vi "Automonous no shift 1 container.vi"() -> ()   [LabVIEW 2014]
uses:
  Autonomous 1 Container with Self Correction.ctl
  2015 Master Code RECYCLE RUSH/2015 Master Code RECYCLE RUSH/Robot Global Data.vi
  Desired Arm Position.vi
  <vilib>/Rock Robotics/WPI/RobotDrive/WPI_RobotDriveGetSetRefNum.vi
panel:
  in  "Cluster":T1
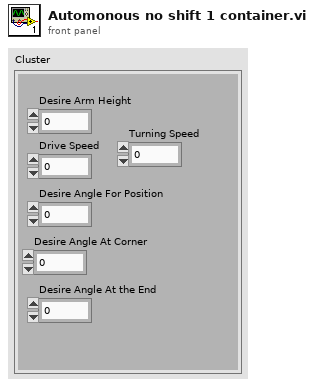
[diagram p1: front panel]
types:
  T1 = cluster{"Desire Arm Height":dbl, "Drive Speed":dbl, "Turning Speed":dbl, "Desire Angle At Corner ":dbl, "Desire Angle At the End":dbl, "Desire Angle For Position":dbl}
  T2 = typedef "Autonomous 1 Container with Self Correction.ctl" = enum16{"Start", "Pick Up Container", "Lift Container", "Drive To S.P", "Drive Straight", "Turn at Corner", "Move to Autozone", "Stop"}
  T3 = typedef "WPI_DigitalInputDevRef.ctl" = cluster{"DevStatus":errorcluster, "DIO Channel":T4, "Controller":T5}
  T4 = typedef "FPGA_DIOChannel.ctl" = enum8{"DIO 0", "DIO 1", "DIO 2", "DIO 3", "DIO 4", "DIO 5", "DIO 6", "DIO 7", "DIO 8", "DIO 9", "DIO MXP 0", "DIO MXP 1", "DIO MXP 2", "DIO MXP 3", "DIO MXP 4", "DIO MXP 5", "DIO MXP 6", "DIO MXP 7", "DIO MXP 8", "DIO MXP 9", "DIO MXP 10", "DIO MXP 11", "DIO MXP 12", "DIO MXP 13", "DIO MXP 14", "DIO MXP 15", "Invalid"}
  T5 = typedef "FPGA_TypedefDigitalModule.ctl" = enum16{"Controller 1"}
  T6 = typedef "WPI_RobotDriveDevRef.ctl" = cluster{"DevStatus":errorcluster, "Motors[]":T7[], "Square Inputs":bool, "Max Output":dbl}
  T7 = typedef "WPI_MotorControlDeviceRef.ctl" = cluster{"DeviceStatus":errorcluster, "Type":T8, "PWM":cluster{"Controller":T5, "PWM Channel":T9, "DeadBand":T10}, "CAN":cluster{"Device Number":u8, "Control Mode":T11, "Semaphore":T12, "Max Vout":dbl, "TalonSRX Control Mode":T13}, "Invert":bool, "TransformRef":T14, "InvTransformRef":T14}
  T8 = typedef "WPI_MotorControlType.ctl" = enum16{"PWM", "CAN", "CANTalonSRX"}
  T9 = typedef "FPGA_DIOPWMChannel.ctl" = enum8{"PWM 0", "PWM 1", "PWM 2", "PWM 3", "PWM 4", "PWM 5", "PWM 6", "PWM 7", "PWM 8", "PWM 9", "PWM MXP 0", "PWM MXP 1", "PWM MXP 2", "PWM MXP 3", "PWM MXP 4", "PWM MXP 5", "PWM MXP 6", "PWM MXP 7", "PWM MXP 8", "PWM MXP 9", "Invalid"}
  T10 = typedef "WPI_PWMDeadband.ctl" = cluster{"Name":string, "maxPositivePwm":i32, "minPositivePwm":i32, "centerPwm":i32, "maxNegativePwm":i32, "minNegativePwm":i32, "angularRange":u16}
  T11 = typedef "WPI_CANJaguar_ControlMode.ctl" = enum8{"Percent VBus", "Current", "Speed", "Position", "Voltage"}
  T12 = typedef "Semaphore RefNum" = refnum<k1>
  T13 = typedef "WPI_CANTalonSRX_APIControlMode.ctl" = enum8{"Percent VBus", "Speed", "Position", "Slave", "Unchanged / Invalid"}
  T14 = typedef "WPI_PWMTransform_ConPane.ctl" = refnum<vi>
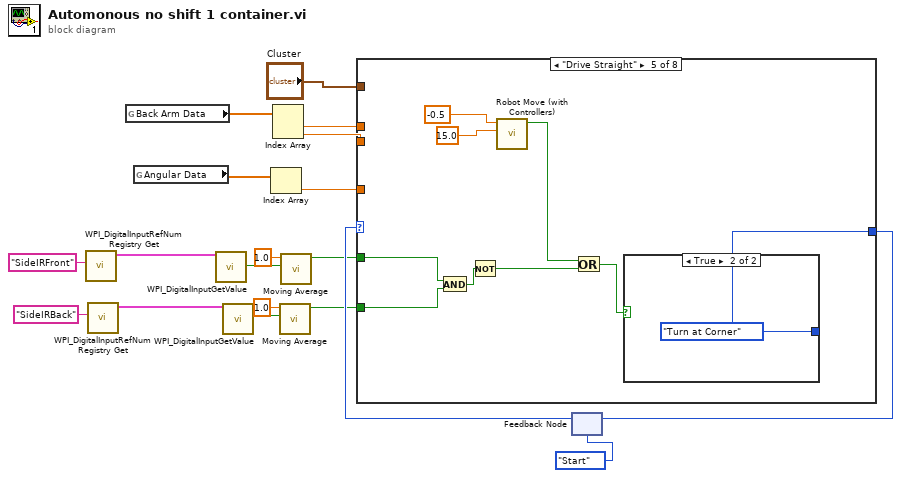
[diagram p0: block diagram]
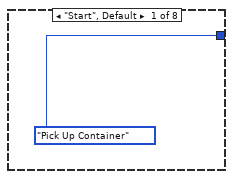
[diagram p2: hidden frame]
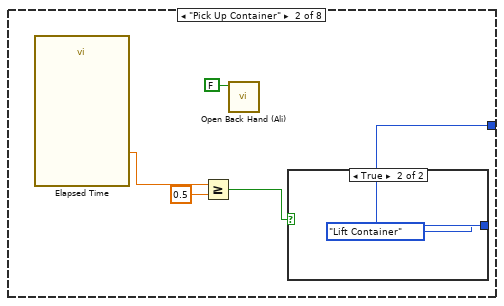
[diagram p3: hidden frame]
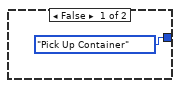
[diagram p4: hidden frame]
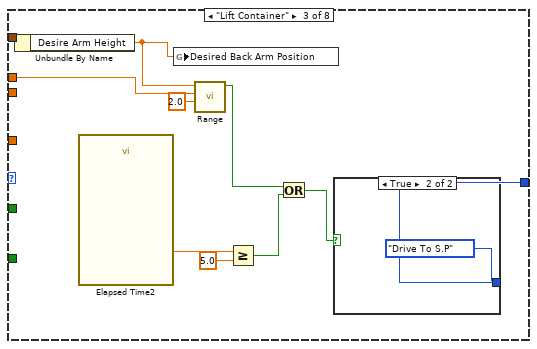
[diagram p5: hidden frame]
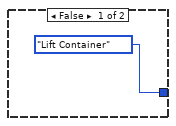
[diagram p6: hidden frame]
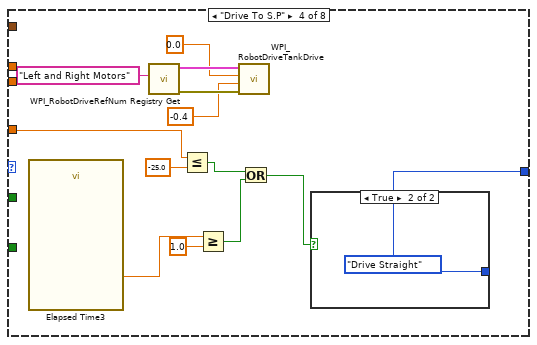
[diagram p7: hidden frame]
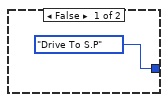
[diagram p8: hidden frame]
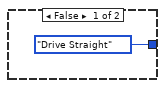
[diagram p9: hidden frame]
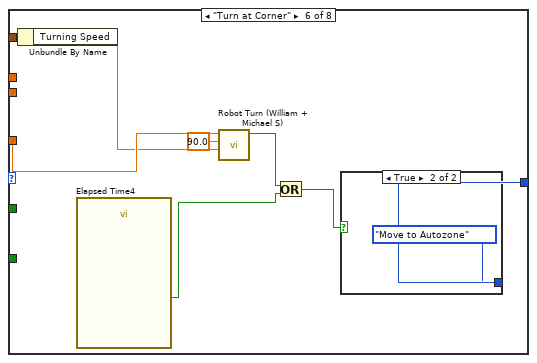
[diagram p10: hidden frame]
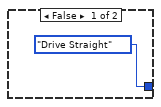
[diagram p11: hidden frame]
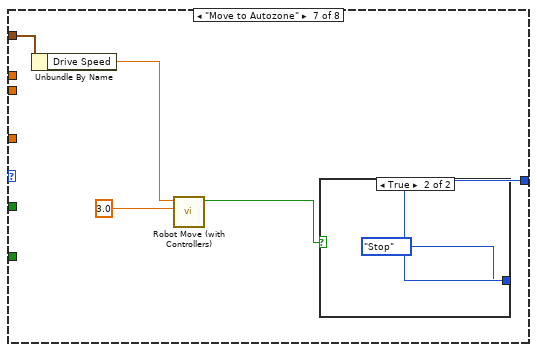
[diagram p12: hidden frame]
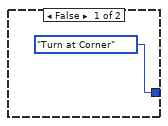
[diagram p13: hidden frame]
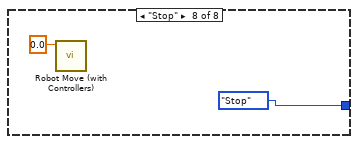
[diagram p14: hidden frame]
diagram:
  n1 = call <vilib>:"WPI_DigitalInputRefNum Registry Get.vi"("refnum name"="SideIRFront") -> ("DigitalInputDevRef"=w5:T3)  [unwired: 9 in, 1 out]
  n2 = call <vilib>:"WPI_DigitalInputRefNum Registry Get.vi"("refnum name"="SideIRBack") -> ("DigitalInputDevRef"=w6:T3)  [unwired: 9 in, 1 out]
  n3 = global read "Robot Global Data.vi" "Back Arm Data"() -> (w16:dbl[])
  n4 = global read "Robot Global Data.vi" "Angular Data"() -> (w12:dbl[])
  n5 = call <vilib>:"WPI_DigitalInputGetValue.vi"("DigitalInputDevRef"=w5) -> ("Value"=w8:bool)  [unwired: 8 in, 2 out]
  n6 = call <vilib>:"WPI_DigitalInputGetValue.vi"("DigitalInputDevRef"=w6) -> ("Value"=w7:bool)  [unwired: 8 in, 2 out]
  n7 = Index Array(array=w12) -> (element=w11:dbl)  [unwired: 1 in]
  n8 = Index Array(array=w16) -> (element #1=w15:dbl, element #2=w14:dbl)  [unwired: 2 in]
  n9 = call "Moving Average.vi"("Value"=w7, "Time Target (s)"=1.0) -> ("Moving Boolean Average"=w3:bool)  [unwired: 9 in]
  n10 = call "Moving Average.vi"("Value"=w8, "Time Target (s)"=1.0) -> ("Moving Boolean Average"=w4:bool)  [unwired: 9 in]
  n11 = feedback #1(Autonomous_1_Container_with_Self_Correction."Start") -> (w18:T2)
  n12 = case shown="\"Drive Straight\"" w18 {
    tunnel: [Autonomous_1_Container_with_Self_Correction."Pick Up Container" w21 w33 w49 w62 w73 w80 Autonomous_1_Container_with_Self_Correction."Stop"] -> w17
    tunnel: w15 -> [_ _ w31 _ _ _ _ _]
    tunnel: w14 -> [_ _ _ _ _ _ _ _]
    tunnel: "Cluster" -> [_ _ w37 _ _ w70 w77 _]
    tunnel: w11 -> [_ _ _ w42 _ w72 _ _]
    tunnel: w4 -> [_ _ _ _ w57 _ _ _]
    tunnel: w3 -> [_ _ _ _ w58 _ _ _]
    frame "Start", Default {
    }
    frame "Pick Up Container" {
      n13 = call "Elapsed Time"() -> ("Elapsed Time (s)"=w24:dbl)  [unwired: 12 in, 7 out]
      n14 = Greater Or Equal?(x=w24, y=0.5) -> (x >= y?=w22:bool)
      n15 = call "Open Back Hand (Ali).vi"("Open?"=FALSE) -> ()  [unwired: 11 in]
      n16 = case shown="True" w22 {
        tunnel: [Autonomous_1_Container_with_Self_Correction."Pick Up Container" Autonomous_1_Container_with_Self_Correction."Lift Container"] -> w21
        frame False {
        }
        frame True {
        }
      }
    }
    frame "Lift Container" {
      n17 = Unbundle By Name(w37) -> ("Desire Arm Height"=w30:dbl)
      n18 = call "Elapsed Time2"() -> ("Elapsed Time (s)"=w36:dbl)  [unwired: 12 in, 7 out]
      n19 = global write "Desired Arm Position.vi" "Desired Back Arm Position"(w30) -> ()
      n20 = call "Range.vi"("Range"=2.0, "Input"=w31, "In Range of"=w30) -> ("In Range?"=w28:bool)  [unwired: 8 in]
      n21 = Greater Or Equal?(x=w36, y=5.0) -> (x >= y?=w34:bool)
      n22 = Or(x=w28, y=w34) -> (x .or. y?=w32:bool)
      n23 = case shown="True" w32 {
        tunnel: [Autonomous_1_Container_with_Self_Correction."Lift Container" Autonomous_1_Container_with_Self_Correction."Drive To S.P"] -> w33
        frame False {
        }
        frame True {
        }
      }
    }
    frame "Drive To S.P" {
      n24 = call "Elapsed Time3"() -> ("Elapsed Time (s)"=w52:dbl)  [unwired: 12 in, 7 out]
      n25 = call <vilib>:"WPI_RobotDriveRefNum Registry Get.vi"("refnum name"="Left and Right Motors") -> ("error out"=w46:errorcluster, "RobotDriveDevRef"=w47:T6)  [unwired: 9 in]
      n26 = Less Or Equal?(x=w42, y=-25.0) -> (x <= y?=w41:bool)
      n27 = Greater Or Equal?(x=w52, y=1.0) -> (x >= y?=w50:bool)
      n28 = call <vilib>:"WPI_RobotDriveTankDrive.vi"("error in (no error)"=w46, "Right axis value"=-0.4, "Left axis value"=0.0, "RobotDriveDevRef"=w47) -> ()  [unwired: 5 in, 3 out]
      n29 = Or(x=w41, y=w50) -> (x .or. y?=w48:bool)
      n30 = case shown="True" w48 {
        tunnel: [Autonomous_1_Container_with_Self_Correction."Drive To S.P" Autonomous_1_Container_with_Self_Correction."Drive Straight"] -> w49
        frame False {
        }
        frame True {
        }
      }
    }
    frame "Drive Straight" {
      n31 = And(x=w57, y=w58) -> (x .and. y?=w56:bool)
      n32 = Not(x=w56) -> (.not. x?=w55:bool)
      n33 = call "Robot Move (with Controllers).vi"("Time Target (s)"=15.0, "Speed"=-0.5) -> ("Stop"=w59:bool)  [unwired: 9 in]
      n34 = Or(x=w59, y=w55) -> (x .or. y?=w63:bool)
      n35 = case shown="True" w63 {
        tunnel: [Autonomous_1_Container_with_Self_Correction."Drive Straight" Autonomous_1_Container_with_Self_Correction."Turn at Corner"] -> w62
        frame False {
        }
        frame True {
        }
      }
    }
    frame "Turn at Corner" {
      n36 = Unbundle By Name(w70) -> ("Turning Speed"=w69:dbl)
      n37 = call "Elapsed Time4"() -> ("Time has Elapsed"=w68:bool)  [unwired: 12 in, 7 out]
      n38 = call "Robot Turn (William + Michael S).vi"("X axis value"=w69, "Desired Degree"=90.0, "Gyro Degrees"=w72) -> ("Stop"=w67:bool)  [unwired: 8 in]
      n39 = Or(x=w67, y=w68) -> (x .or. y?=w66:bool)
      n40 = case shown="True" w66 {
        tunnel: [Autonomous_1_Container_with_Self_Correction."Drive Straight" Autonomous_1_Container_with_Self_Correction."Move to Autozone"] -> w73
        frame False {
        }
        frame True {
        }
      }
    }
    frame "Move to Autozone" {
      n41 = Unbundle By Name(w77) -> ("Drive Speed"=w76:dbl)
      n42 = call "Robot Move (with Controllers).vi"("Time Target (s)"=3.0, "Speed"=w76) -> ("Stop"=w79:bool)  [unwired: 9 in]
      n43 = case shown="True" w79 {
        tunnel: [Autonomous_1_Container_with_Self_Correction."Turn at Corner" Autonomous_1_Container_with_Self_Correction."Stop"] -> w80
        frame False {
        }
        frame True {
        }
      }
    }
    frame "Stop" {
      n44 = call "Robot Move (with Controllers).vi"("Speed"=0.0) -> ()  [unwired: 10 in, 1 out]
    }
  }
  n45 = feedback-in #1(w17) -> ()
